vi "for-loop.vi"() -> ()   [LabVIEW 2025]
panel:
  out "sum":i32
  out "Array":dbl[](array[numeric])
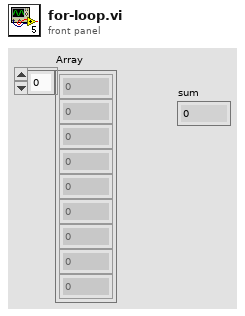
[diagram p1: front panel]
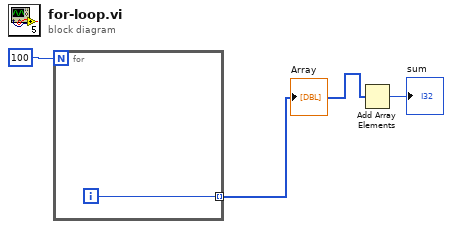
[diagram p0: block diagram]
diagram:
  n1 = for {
    N: 100 -> [_]
    tunnel: [w4] -> w2 mode=indexing
    i -> [w4]
  }
  "Array" <- w2
  n2 = Add Array Elements(numeric array=w2) -> (sum=→"sum":i32)
